vi "removeDuplicatesFromArray.vi"(8 "error in (no error)":errorcluster, 10 "Array":variant[](array[variant]), 11 "ScriptEventList in":refnum<class "ScriptEventList.lvclass">) -> (0 "error out":errorcluster, 2 "Array out":variant[](array[variant]), 3 "ScriptEventList out":refnum<class "ScriptEventList.lvclass">)   [LabVIEW 2009, in "Tools.lvlib" / "Scripting.lvlib" / "ScriptEventList.lvclass"]
uses:
  ScriptEventList.lvclass
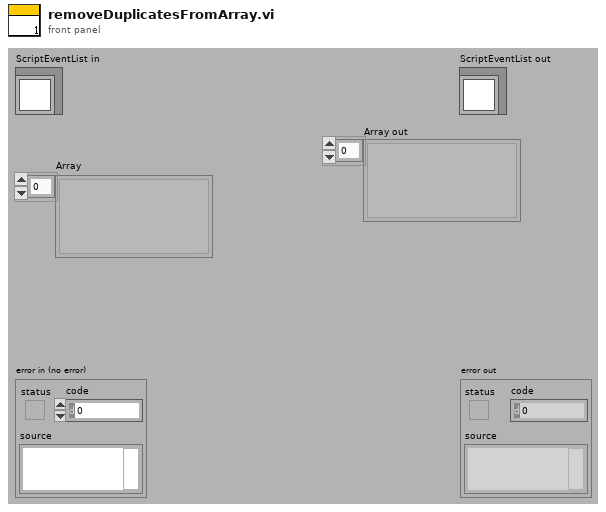
[diagram p1: front panel]
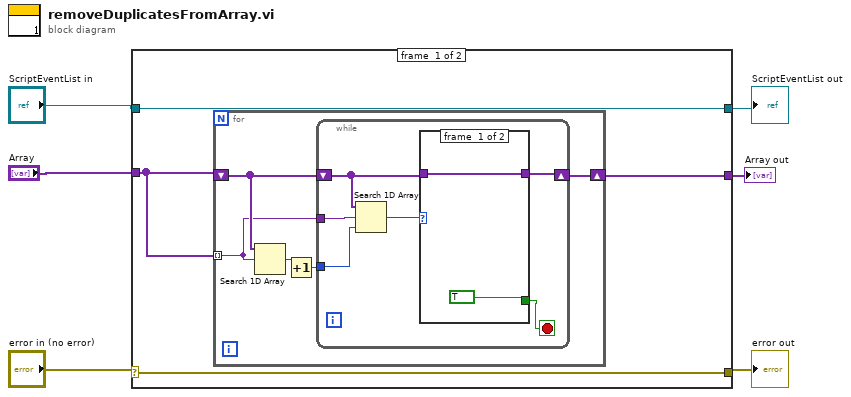
[diagram p0: block diagram]
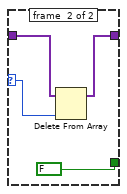
[diagram p2: hidden frame]
diagram:
  n1 = case shown="No Error" "error in (no error)" {
    selector: "error in (no error)" -> [w9 w29]
    tunnel: [w9 w29] -> w4
    tunnel: [w10 w28] -> w5
    tunnel: "ScriptEventList in" -> [w10 w28]
    tunnel: "Array" -> [w8 _]
    tunnel: [w7 _] -> w2
    frame #0 {
      n2 = for {
        shift-right: [w15] -> w7
        shift-left: w8 -> [w12]
        tunnel: w8 -> [w11] mode=indexing
        n3 = Search 1D Array(1D array=w12, element=w11) -> (index of element=w14:i32)  [unwired: 1 in]
        n4 = Increment(x=w14) -> (x+1=w13:i32)
        n5 = while {
          shift-right: [w19] -> w15
          shift-left: w12 -> [w17]
          tunnel: w13 -> [w18]
          tunnel: w11 -> [w16]
          stop <- w20 stop-if-true
          n6 = Search 1D Array(1D array=w17, element=w16, start index (0)=w18) -> (index of element=w21:i32)
          n7 = case shown="Default" w21 {
            selector: w21 -> [_ w26]
            tunnel: [TRUE FALSE] -> w20
            tunnel: w17 -> [w22 w25]
            tunnel: [w22 w24] -> w19
            frame #0 {
            }
            frame #1 {
              n8 = Delete From Array(array=w25, index=w26) -> (array with subset deleted=w24:variant[])  [unwired: 1 in, 1 out]
            }
          }
        }
      }
    }
    frame #1 {
    }
  }
  "error out" <- w4
  "ScriptEventList out" <- w5
  "Array out" <- w2
